vi "Write File.vi"(7 "index":i32, 8 "error in":errorcluster, 9 "Money":string, 11 "Account Details":T1(array[cluster])=[{"Account"="12345", "First"="Amol", "Last"="Jadhav", "Money"="100000"}, {"Account"="23456", "First"="Prashant", "Last"="Kumar", "Money"="Singh"}, {"Account"="34567", "First"="Bryan", "Last"="Smith", "Money"="800"}, {"Account"="45678", "First"="Julie", "Last"="Ramirez", "Money"="46000"}]) -> (0 "error out":errorcluster)   [LabVIEW 2019, in "SubVI.lvlib"]
uses:
  <vilib>/Utility/file.llb/Write Delimited Spreadsheet (string).vi
  SubVIs/SubVI.lvlib
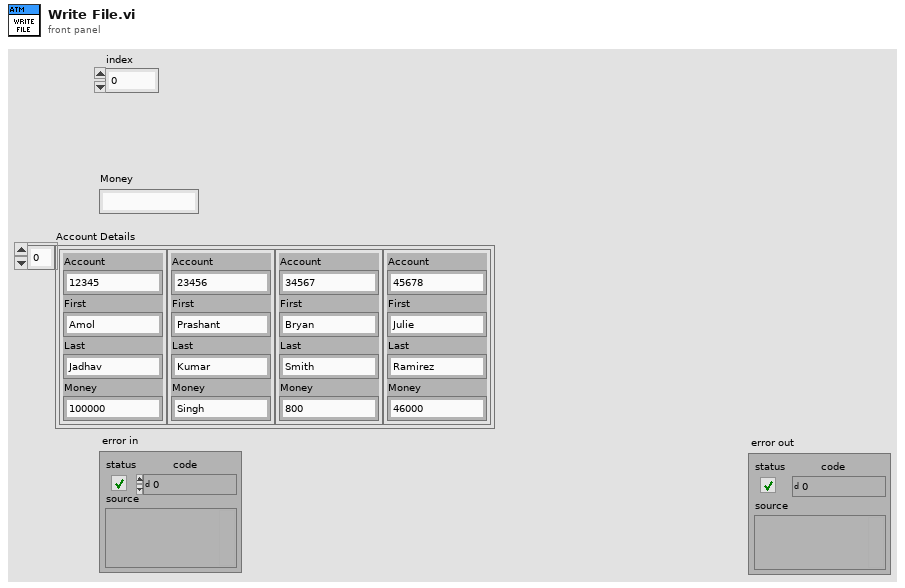
[diagram p1: front panel]
types:
  T1 = cluster{"Account":string, "First":string, "Last":string, "Money":string}[]
  T2 = cluster{"Account":string, "First":string, "Last":string, "Money":string}
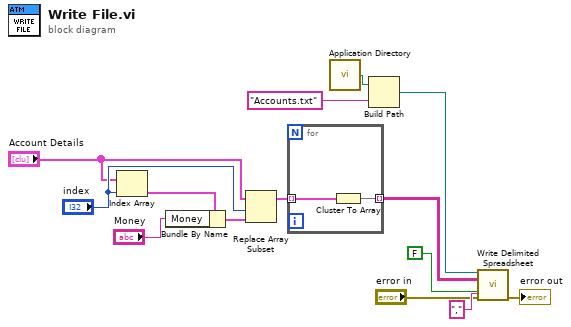
[diagram p0: block diagram]
diagram:
  n1 = Index Array(array="Account Details", index="index") -> (element=w3:T2)
  n2 = Bundle By Name(cluster=w3, "Money"="Money") -> (w5:T2)
  n3 = Replace Array Subset(array="Account Details", new element=w5, index="index") -> (w8:T1)
  n4 = for {
    tunnel: w8 -> [w15] mode=indexing
    tunnel: [w16] -> w2 mode=indexing
    n5 = Cluster To Array(cluster=w15) -> (array=w16:string[])
  }
  n6 = call <vilib>:"Application Directory.vi"() -> ("Application Directory"=w14:path)
  n7 = Build Path(base path=w14, name or relative path="Accounts.txt") -> (appended path=w12:path)
  n8 = call-poly <vilib>:"Write Delimited Spreadsheet.vi"("file path (dialog if empty)"=w12, "2D data"=w2, "append to file? (new file:F)"=FALSE, "error in (no error)"="error in", "delimiter (\\t)"="," ("delimiter (\\t)")) -> ("error out"=→"error out":errorcluster)  [unwired: 9 in, 1 out]
